vi "Get Data Type Name.vi"(11 "String Type View in":refnum<class "Integer Type View.lvclass">) -> (3 "Data Type Name":string="Default Data Type")   [LabVIEW 2017, in "Integer Type View.lvclass"]
uses:
  <vilib>/gpm_packages/@cs/Test-executive-builder/Source/Test Executive Builder Dialogs/Integer Type View/Integer Type View.lvclass
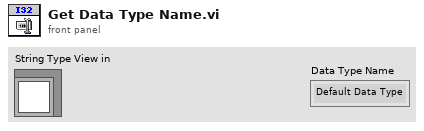
[diagram p1: front panel]
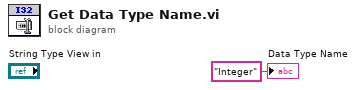
[diagram p0: block diagram]
diagram:
  "Data Type Name" <- "Integer" ("Data Type Name")
